vi "PPSU data getter.vi"(0 "data in":string, 11 "error in":errorcluster) -> (3 "FAULT":T1, 4 "Voltage PPSU":string, 6 "Current PPSU":string, 8 "Fault":string, 10 "status":string, 14 "STATUS":T1, 15 "error in  2":errorcluster)   [LabVIEW 2022 SP3]
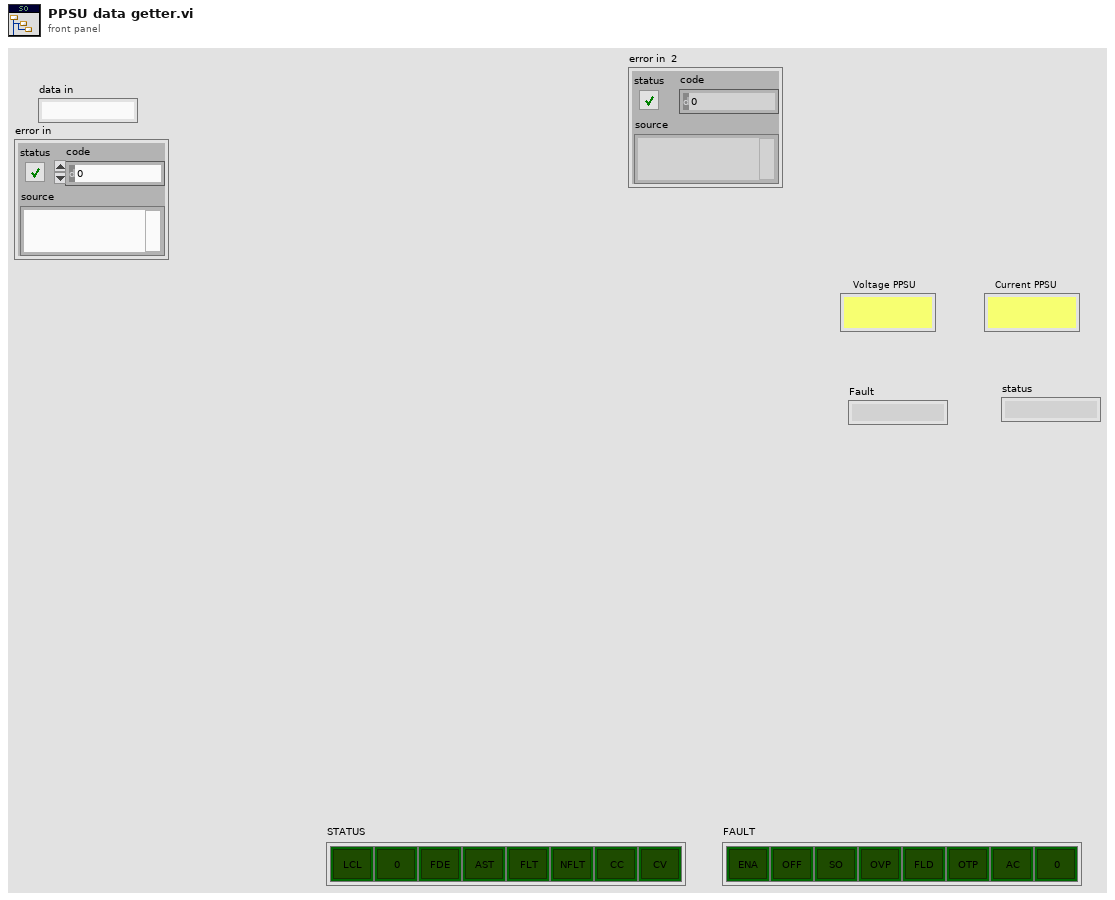
[diagram p1: front panel]
types:
  T1 = cluster{"[0]":bool, "[1]":bool, "[2]":bool, "[3]":bool, "[4]":bool, "[5]":bool, "[6]":bool, "[7]":bool, "[8]":bool}
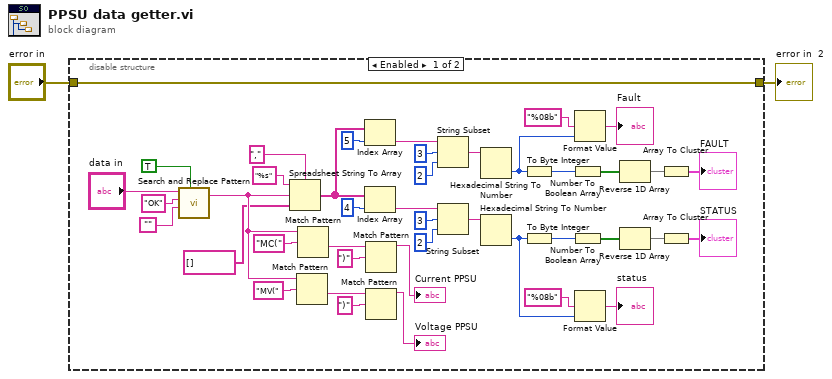
[diagram p0: block diagram]
diagram:
  n1 = disable-structure shown="Enabled" {
    disable-tunnel: [w4 _] -> w2
    disable-tunnel: "error in" -> [w4 _]
    frame Enabled {
      n2 = call <vilib>:"Search and Replace Pattern.vi"("string"="data in", "regular expression (\"\")"="OK" ("regular expression (\"\")"), "replace string (\"\")"="" ("replace string (\"\")"), "replace all? (F)"=TRUE) -> ("result string"=w36:string)  [unwired: 1 in, 1 out]
      n3 = Spreadsheet String To Array(delimiter (Tab)=",", format string="%s", spreadsheet string=w36, array type (2D Dbl)=string[] []) -> (array=w35:string[])
      n4 = Match Pattern(string=w36, regular expression="MV(") -> (after substring=w41:string)  [unwired: 1 in, 3 out]
      n5 = Match Pattern(string=w36, regular expression="MC(") -> (after substring=w32:string)  [unwired: 1 in, 3 out]
      n6 = Index Array(array=w35, index=5) -> (element=w6:string)
      n7 = Index Array(array=w35, index=4) -> (element=w12:string)
      n8 = Match Pattern(string=w32, regular expression=")") -> (before substring=→"Current PPSU":string)  [unwired: 1 in, 3 out]
      n9 = Match Pattern(string=w41, regular expression=")") -> (before substring=→"Voltage PPSU":string)  [unwired: 1 in, 3 out]
      n10 = String Subset(string=w6, offset (0)=3, length (rest)=2 ("length (rest)")) -> (substring=w8:string)
      n11 = String Subset(string=w12, offset (0)=3, length (rest)=2 ("length (rest)")) -> (substring=w16:string)
      n12 = Hexadecimal String To Number(string=w8) -> (number=w11:u32)  [unwired: 2 in, 1 out]
      n13 = Hexadecimal String To Number(string=w16) -> (number=w13:u32)  [unwired: 2 in, 1 out]
      n14 = To Byte Integer(number=w11) -> (8bit integer=w7:i8)
      n15 = To Byte Integer(number=w13) -> (8bit integer=w17:i8)
      n16 = Number To Boolean Array(number=w7) -> (Boolean array=w10:bool[])
      n17 = Number To Boolean Array(number=w17) -> (Boolean array=w14:bool[])
      n18 = Format Value(format string="%08b", value (0)=w11) -> (output string=→"Fault":string)  [unwired: 1 in]
      n19 = Format Value(format string="%08b", value (0)=w13) -> (output string=→"status":string)  [unwired: 1 in]
      n20 = Reverse 1D Array(array=w10) -> (reversed array=w9:bool[])
      n21 = Reverse 1D Array(array=w14) -> (reversed array=w15:bool[])
      n22 = Array To Cluster(array=w9) -> (cluster=→"FAULT":T1)
      n23 = Array To Cluster(array=w15) -> (cluster=→"STATUS":T1)
    }
    frame Disabled {
    }
  }
  "error in  2" <- w2
